vi "Update Add Channel.vi"(4 "Area Height":u32, 5 "Display State In":T4={"Current Channels Info"=[], "Help Prefix"="", "Max Display Size"=8, "Max Size"=8, "Show Buttons"=TRUE, "Data Valid"=refnum, "Show Range"=FALSE, "Range Items"=[], "Range Index"=[]} caption="State", 6 "Number of Row":i32, 7 "Channels In":T1, 8 "error in (no error)":errorcluster, 11 "Add Channel Reference":refnum<vi>) -> (0 "error out":errorcluster)   [LabVIEW 2021, in "myRIO Channel List.xctl"]
uses:
  <vilib>/myRIO/Common/Express VI Framework/xctls/myRIO Channel List/myRIO Channel List.xctl
  <vilib>/myRIO/Common/Express VI Framework/xctls/myRIO Channel List/State.ctl
  <vilib>/myRIO/Common/Profile Manager Framework/typedefs/Channel Info.ctl
  <vilib>/myRIO/Common/Express VI Framework/typedefs/Data Validate Ref.ctl
  <vilib>/myRIO/Common/Express VI Framework/xctls/myRIO Channel List/Data.ctl
  <vilib>/myRIO/Common/Express VI Framework/xctls/myRIO Channel List/typedefs/Channel Data.ctl
  <vilib>/myRIO/Common/Express VI Framework/xctls/myRIO Channel List/typedefs/Remove Channel.ctl
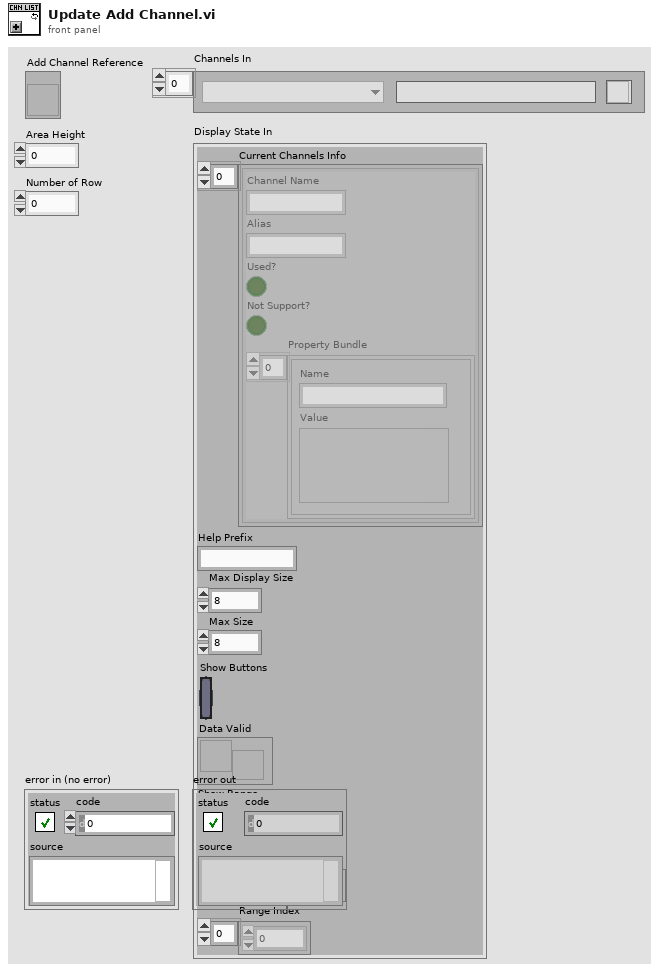
[diagram p1: front panel]
types:
  T1 = typedef "myRIO Channel List.xctl/Data.ctl" = T2[]
  T2 = typedef "myRIO Channel List.xctl/Channel Data.ctl" = cluster{"Channel Name":u16, "Channel Alias":string, "Remove Channel":T3, "Index":i32}
  T3 = typedef "myRIO Channel List.xctl/Remove Channel.ctl" = bool
  T4 = typedef "myRIO Channel List.xctl/State.ctl" = cluster{"Current Channels Info":T5[], "Help Prefix":string, "Max Display Size":i32, "Max Size":i32, "Show Buttons":bool, "Data Valid":T6, "Show Range":bool, "Range Items":string[], "Range Index":i32[]}
  T5 = typedef "Channel Info.ctl" = cluster{"Channel Name":string, "Alias":string, "Used?":bool, "Not Support?":bool, "Property Bundle":cluster{"Name":string, "Value":variant}[]}
  T6 = typedef "Data Validate Ref.ctl" = refnum<user-event>
  T7 = enum8{"Enabled", "Disabled", "Disabled and Grayed Out"}
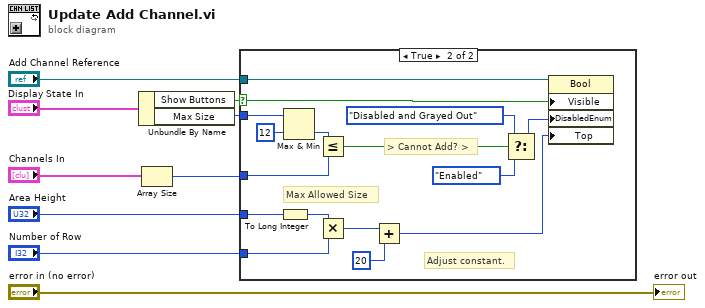
[diagram p0: block diagram]
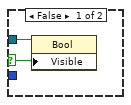
[diagram p2: hidden frame]
diagram:
  n1 = Unbundle By Name("Display State In") -> ("Show Buttons"=w5:bool, "Max Size"=w8:i32)
  n2 = Array Size(array="Channels In") -> (size(s)=w7:i32)
  n3 = case shown="True" w5 {
    selector: w5 -> [w10 w23]
    tunnel: w8 -> [_ w19]
    tunnel: w7 -> [_ w18]
    tunnel: "Add Channel Reference" -> [w11 w25]
    tunnel: "Area Height" -> [_ w17]
    tunnel: "Number of Row" -> [_ w16]
    frame False {
      n4 = property class="Bool"(reference=w11, "Visible"=w10) -> ()  [unwired: 1 in, 2 out]
    }
    frame True {
      # "> Cannot Add? >"
      # "Adjust constant."
      # "Max Allowed Size"
      n5 = To Long Integer(number=w17) -> (32bit integer=w15:i32)
      n6 = Max & Min(x=w19, y=12 ("Max Allowed Size")) -> (min(x,y)=w26:i32)  [unwired: 1 out]
      n7 = Less Or Equal?(x=w26, y=w18) -> (x <= y?=w24:bool)
      n8 = Multiply(x=w15, y=w16) -> (x*y=w13:i32)
      n9 = Add(x=w13, y=20) -> (x+y=w14:i32)
      n10 = Select(t=T7."Disabled and Grayed Out" ("Disabled"), s=w24, f=T7."Enabled" ("Disabled")) -> (s? t:f=w20:T7)
      n11 = property class="Bool"(reference=w25, "Visible"=w23, "DisabledEnum"=w20, "Top"=w14) -> ()  [unwired: 1 in, 2 out]
    }
  }
  "error out" <- "error in (no error)"
